vi "Background_task_in_a_Class.vi"() -> ()   [LabVIEW 2014]
uses:
  scr/axopatch-200B/axopatch-200B.lvclass
panel:
  out "branching test":dbl
  out "test 2":dbl
  out "test":dbl
  out "x+y":dbl
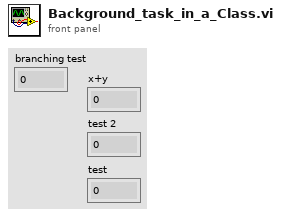
[diagram p1: front panel]
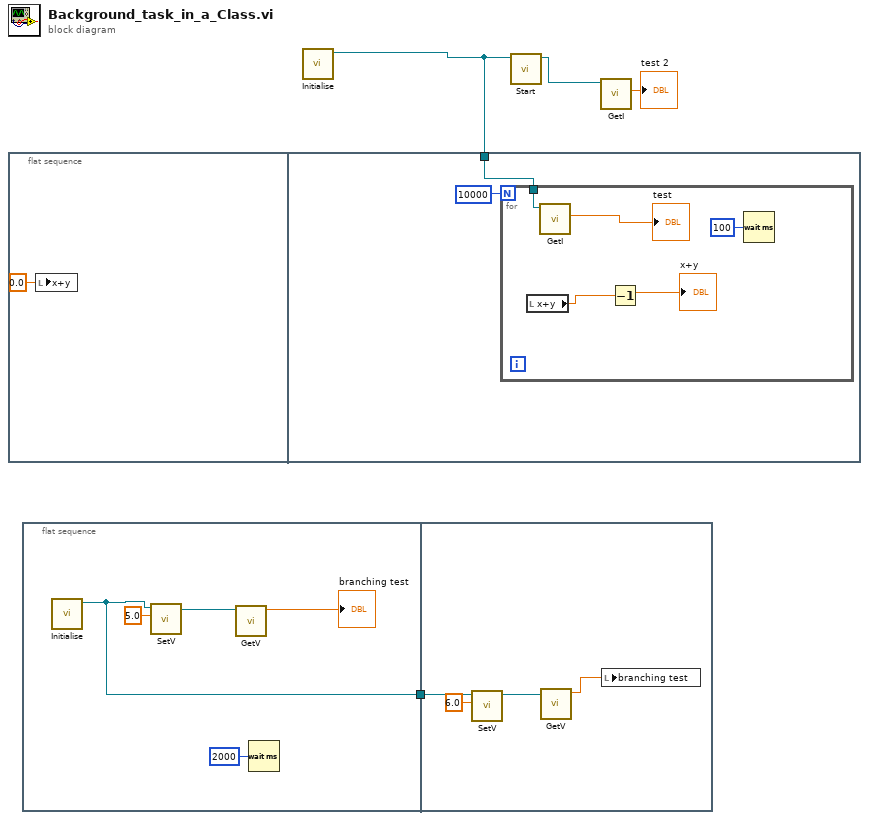
[diagram p0: block diagram]
diagram:
  n1 = flat-sequence {
    tunnel: w1 -> [w6]
    frame #0 {
      n2 = local write "x+y"(0.0 ("x+y")) -> ()
    }
    frame #1 {
      n3 = for {
        N: 10000 -> [_]
        tunnel: w6 -> [w8]
        n4 = local read "x+y"() -> (w11:dbl)
        n5 = call "GetI.vi"("axopatch-200B in"=w8) -> ("test"=→"test":dbl)  [unwired: 9 in, 1 out]
        n6 = Decrement(x=w11) -> (x-1=→"x+y":dbl)
        n7 = Wait (ms)(milliseconds to wait=u32 100) -> ()  [unwired: 1 out]
      }
    }
  }
  n8 = flat-sequence {
    tunnel: [w14] -> w2
    tunnel: w2 -> [w21]
    frame #0 {
      n9 = call "Initialise.vi"() -> ("axopatch-200B out"=w14:refnum<class "axopatch-200B.lvclass">)  [unwired: 10 in, 1 out]
      n10 = call "SetV.vi"("test"=5.0, "axopatch-200B in"=w14) -> ("axopatch-200B out"=w16:refnum<class "axopatch-200B.lvclass">)  [unwired: 8 in, 1 out]
      n11 = call "GetV.vi"("axopatch-200B in"=w16) -> ("test"=→"branching test":dbl)  [unwired: 9 in, 1 out]
      n12 = Wait (ms)(milliseconds to wait=u32 2000) -> ()  [unwired: 1 out]
    }
    frame #1 {
      n13 = call "SetV.vi"("test"=6.0, "axopatch-200B in"=w21) -> ("axopatch-200B out"=w20:refnum<class "axopatch-200B.lvclass">)  [unwired: 8 in, 1 out]
      n14 = call "GetV.vi"("axopatch-200B in"=w20) -> ("test"=w18:dbl)  [unwired: 9 in, 1 out]
      n15 = local write "branching test"(w18) -> ()
    }
  }
  n16 = call "Initialise.vi"() -> ("axopatch-200B out"=w1:refnum<class "axopatch-200B.lvclass">)  [unwired: 10 in, 1 out]
  n17 = call "Start.vi"("axopatch-200B in"=w1) -> ("axopatch-200B in 2"=w4:refnum<class "axopatch-200B.lvclass">)  [unwired: 10 in]
  n18 = call "GetI.vi"("axopatch-200B in"=w4) -> ("test"=→"test 2":dbl)  [unwired: 9 in, 1 out]
